vi "Create Engine Folder and Copy RT Template.vi"(8 "error in":errorcluster, 9 "Project Root":path, 10 "Project Name":string, 11 "Inline-Async":refnum<class "NIVS_Inline HW Interface (Inline-Async).lvclass">) -> (0 "error out":errorcluster)   [LabVIEW 2020, in "NIVS_Inline HW Interface (Inline-Async).lvclass"]
uses:
  NIVS_Inline HW Interface (Inline-Async).lvclass
  C:/dev/Karthick/FPGA Addons Packages/niveristand-custom-device-wizard/ProjectTemplate/Source/NI VeriStand/Custom Device/Template Classes/NIVS_CD Template/NIVS_CD Template.lvclass
  NIVS_Consolidated_CDW_MetaDataObj/CD Engine lvlib.ctl
  NIVS_Consolidated_CDW_MetaDataObj/Common.ctl
  NIVS_CD Template/NIVS_CD Template.lvclass/NIVS_CD Template.ctl
  NIVS_Consolidated_CDW_MetaDataObj/Common.vi
  NIVS_Consolidated_CDW_MetaDataObj/NIVS_Consolidated_CDW_MetaDataObj.lvclass
  NIVS_CD Template/NIVS_CD Template.lvclass
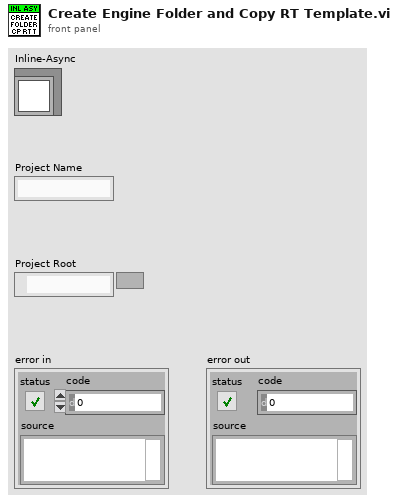
[diagram p1: front panel]
types:
  T1 = typedef "NIVS_Consolidated_CDW_MetaDataObj.lvclass/Common.ctl" = enum16{"ProjectName", "TemplatesFolderName", "PPLTemplatesFolderName", "ProjectTemplatePathAndName", "ProjectPPLTemplatePathAndName", "TimingAndSyncFolderName", "CustomDeviceFolderName", "PathToTemplates", "PathToPPLTemplates", "PathToExplorerPPLTemplates", "PathToEnginePPLTemplates", "PathToConfigurationFile", "ProjectConfigurationName"}
  T2 = typedef "NIVS_Consolidated_CDW_MetaDataObj.lvclass/CD Engine lvlib.ctl" = enum16{"LibraryFileName", "LibraryFolderName", "Engine.FolderName", "Engine.Init.FolderName", "Engine.Run.FolderName", "Engine.Shutdown.FolderName", "Types.FolderName", "Engine.RT Driver VI.TemplatePath", "Engine.RT Driver VI.FileName", "Engine.PPL.RT Driver VI_InlineAsync.FileName", "Engine.RTStateVariables.Name", "Engine.PPL.RTStateVariables.Name", "Engine.RTStateVariables.Name.NoExtension", "Engine.Async.NameExtension", "Engine.Async.TemplateName", "Engine.PPL.Async.TemplateName", "Engine.PPL.Async.InitVSGlobals.Name", "Engine.PPL.RT Driver VI_Inline.FileName", "Engine.LaunchCommandLoop.Name", "Engine.CommandLoop.Name"}
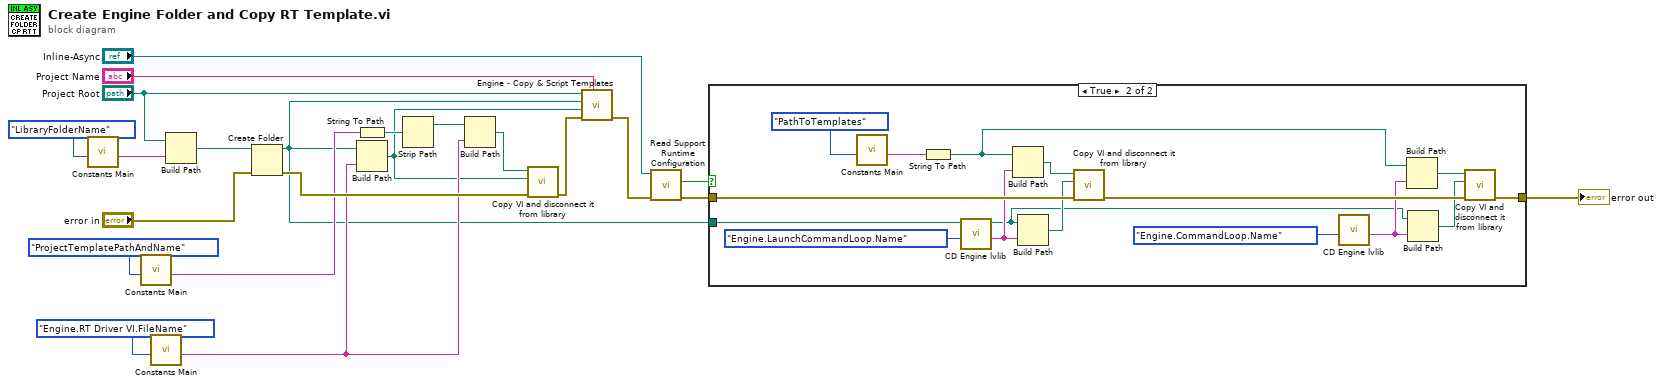
[diagram p0: block diagram]
diagram:
  n1 = call-poly "Constants Main.vi"("Action"=CD_Engine_lvlib."LibraryFolderName") -> ("Output"=w7:string)  [unwired: 10 in]
  n2 = call-poly "Constants Main.vi"("Action"=Common."ProjectTemplatePathAndName") -> ("Output"=w11:string)  [unwired: 10 in]
  n3 = call-poly "Constants Main.vi"("Action"=CD_Engine_lvlib."Engine.RT Driver VI.FileName") -> ("Output"=w12:string)  [unwired: 10 in]
  n4 = Build Path(base path="Project Root", name or relative path=w7) -> (appended path=w5:path)
  n5 = Create Folder(path (use dialog)=w5, error in="error in") -> (created path=w1:path, error out=w22:errorcluster)  [unwired: 1 in, 1 out]
  n6 = String To Path(string=w11) -> (path=w10:path)
  n7 = Build Path(base path=w1, name or relative path=w12) -> (appended path=w2:path)
  n8 = Strip Path(path=w10) -> (stripped path=w14:path)  [unwired: 1 out]
  n9 = Build Path(base path=w14, name or relative path=w12) -> (appended path=w9:path)
  n10 = call "Copy VI and disconnect it from library.vi"("error in (no error)"=w22, "VI Target Path"=w2, "VI Source Path"=w9) -> ("error out"=w20:errorcluster)  [unwired: 8 in]
  n11 = call "Engine - Copy & Script Templates.vi"("CD Name"="Project Name", "error in (no error)"=w20, "RT Driver VI Path"=w2, "RT Driver Folder Path"=w1, "CD Source Folder Path"="Project Root") -> ("error out"=w19:errorcluster)  [unwired: 6 in]
  n12 = call "Read Support Runtime Configuration.vi"("error in"=w19, "NIVS_CD Template in"="Inline-Async") -> ("error out"=w18:errorcluster, "Support Runtime Configuration"=w3:bool)  [unwired: 7 in, 1 out]
  n13 = case shown="True" w3 {
    tunnel: [w23 w37] -> w17
    tunnel: w18 -> [w23 w36]
    tunnel: w1 -> [_ w24]
    frame False {
    }
    frame True {
      n14 = call-poly "Constants Main.vi"("Action"=Common."PathToTemplates") -> ("Output"=w31:string)  [unwired: 10 in]
      n15 = String To Path(string=w31) -> (path=w26:path)
      n16 = call "CD Engine lvlib.vi"("Action"=CD_Engine_lvlib."Engine.LaunchCommandLoop.Name") -> ("Output"=w30:string)  [unwired: 10 in]
      n17 = Build Path(base path=w26, name or relative path=w30) -> (appended path=w32:path)
      n18 = Build Path(base path=w24, name or relative path=w30) -> (appended path=w34:path)
      n19 = call "Copy VI and disconnect it from library.vi"("error in (no error)"=w36, "VI Target Path"=w34, "VI Source Path"=w32) -> ("error out"=w38:errorcluster)  [unwired: 8 in]
      n20 = call "CD Engine lvlib.vi"("Action"=CD_Engine_lvlib."Engine.CommandLoop.Name") -> ("Output"=w25:string)  [unwired: 10 in]
      n21 = Build Path(base path=w26, name or relative path=w25) -> (appended path=w27:path)
      n22 = Build Path(base path=w24, name or relative path=w25) -> (appended path=w28:path)
      n23 = call "Copy VI and disconnect it from library.vi"("error in (no error)"=w38, "VI Target Path"=w28, "VI Source Path"=w27) -> ("error out"=w37:errorcluster)  [unwired: 8 in]
    }
  }
  "error out" <- w17
